vi "OpenCamera.vi"(8 "error in (no error)":errorcluster, 10 "Camera ID":string, 11 "ZWO_ASI in":refnum<class "ZWO_ASI.lvclass">) -> (0 "error out":errorcluster, 3 "ZWO_ASI out":refnum<class "ZWO_ASI.lvclass">)   [LabVIEW 2023, in "ZWO_ASI.lvlib" / "ZWO_ASI.lvclass"]
uses:
  ZWO_ASI.lvclass
  ZWO_ASI.lvclass/ZWO_ASI.ctl
  <userlib>/ASICamera2_no_err/ASICamera2_no_err.lvlib
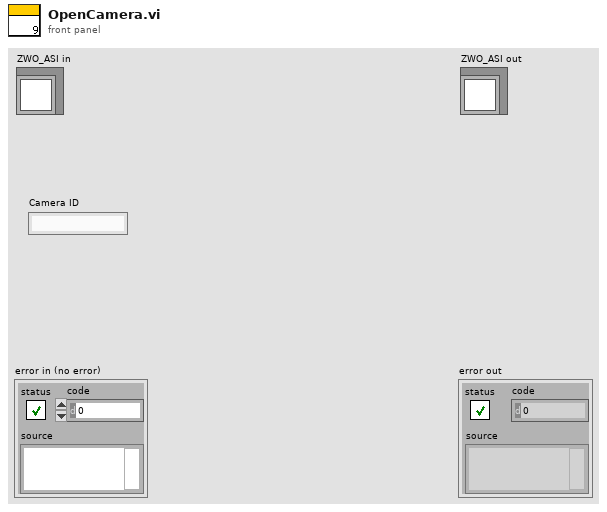
[diagram p1: front panel]
types:
  T1 = cluster{"Name[0]":i8, "Name[1]":i8, "Name[2]":i8, "Name[3]":i8, "Name[4]":i8, "Name[5]":i8, "Name[6]":i8, "Name[7]":i8, "Name[8]":i8, "Name[9]":i8, "Name[10]":i8, "Name[11]":i8, "Name[12]":i8, "Name[13]":i8, "Name[14]":i8, "Name[15]":i8, "Name[16]":i8, "Name[17]":i8, "Name[18]":i8, "Name[19]":i8, "Name[20]":i8, "Name[21]":i8, "Name[22]":i8, "Name[23]":i8, "Name[24]":i8, "Name[25]":i8, "Name[26]":i8, "Name[27]":i8, "Name[28]":i8, "Name[29]":i8, "Name[30]":i8, "Name[31]":i8, "Name[32]":i8, "Name[33]":i8, "Name[34]":i8, "Name[35]":i8, "Name[36]":i8, "Name[37]":i8, "Name[38]":i8, "Name[39]":i8, "Name[40]":i8, "Name[41]":i8, "Name[42]":i8, "Name[43]":i8, "Name[44]":i8, "Name[45]":i8, "Name[46]":i8, "Name[47]":i8, "Name[48]":i8, "Name[49]":i8, "Name[50]":i8, "Name[51]":i8, "Name[52]":i8, "Name[53]":i8, "Name[54]":i8, "Name[55]":i8, "Name[56]":i8, "Name[57]":i8, "Name[58]":i8, "Name[59]":i8, "Name[60]":i8, "Name[61]":i8, "Name[62]":i8, "Name[63]":i8, "CameraID":i32, "MaxHeight":i32, "MaxWidth":i32, "IsColorCam":u32, "BayerPattern":u32, "SupportedBins[0]":i32, "SupportedBins[1]":i32, "SupportedBins[2]":i32, "SupportedBins[3]":i32, "SupportedBins[4]":i32, "SupportedBins[5]":i32, "SupportedBins[6]":i32, "SupportedBins[7]":i32, "SupportedBins[8]":i32, "SupportedBins[9]":i32, "SupportedBins[10]":i32, "SupportedBins[11]":i32, "SupportedBins[12]":i32, "SupportedBins[13]":i32, "SupportedBins[14]":i32, "SupportedBins[15]":i32, "SupportedVideoFormat[0]":u32, "SupportedVideoFormat[1]":u32, "SupportedVideoFormat[2]":u32, "SupportedVideoFormat[3]":u32, "SupportedVideoFormat[4]":u32, "SupportedVideoFormat[5]":u32, "SupportedVideoFormat[6]":u32, "SupportedVideoFormat[7]":u32, "@dummy control@":i8, "@dummy control@":i8, "@dummy control@":i8, "@dummy control@":i8, "PixelSize":dbl, "MechanicalShutter":u32, "ST4Port":u32, "IsCoolerCam":u32, "IsUSB3Host":u32, "IsUSB3Camera":u32, "ElecPerADU":sgl, "Unused[0]":i8, "Unused[1]":i8, "Unused[2]":i8, "Unused[3]":i8, "Unused[4]":i8, "Unused[5]":i8, "Unused[6]":i8, "Unused[7]":i8, "Unused[8]":i8, "Unused[9]":i8, "Unused[10]":i8, "Unused[11]":i8, "Unused[12]":i8, "Unused[13]":i8, "Unused[14]":i8, "Unused[15]":i8, "Unused[16]":i8, "Unused[17]":i8, "Unused[18]":i8, "Unused[19]":i8, "Unused[20]":i8, "Unused[21]":i8, "Unused[22]":i8, "Unused[23]":i8}
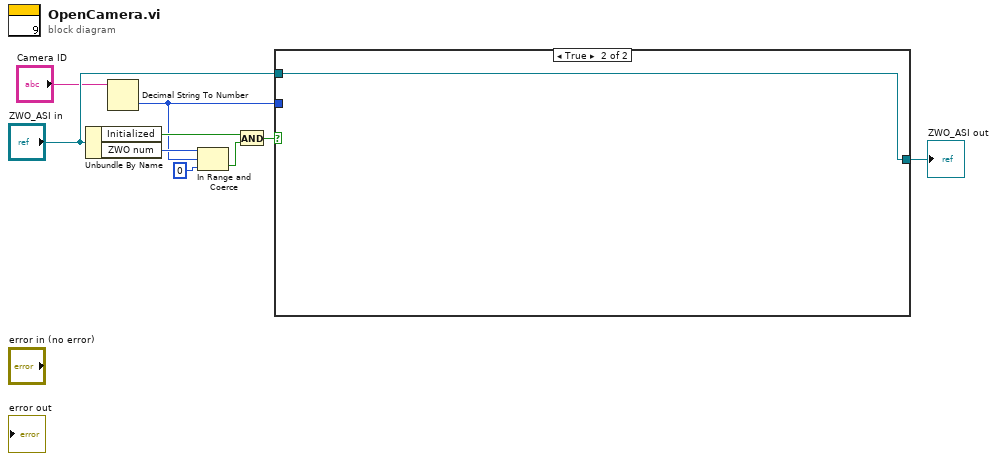
[diagram p0: block diagram]
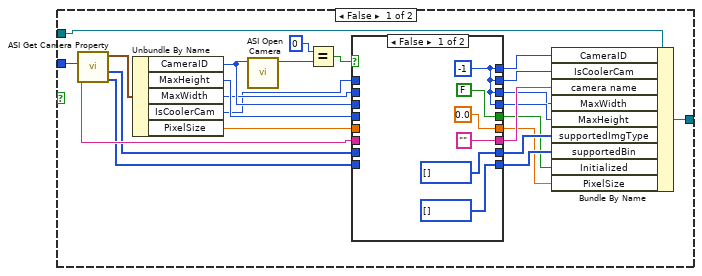
[diagram p2: hidden frame]
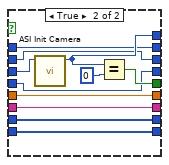
[diagram p3: hidden frame]
diagram:
  n1 = Unbundle By Name("ZWO_ASI in") -> ("Initialized"=w3:bool, "ZWO num"=w6:i32)
  n2 = Decimal String To Number(string="Camera ID") -> (number=w1:i32)  [unwired: 2 in, 1 out]
  n3 = In Range and Coerce(upper limit=w6, x=w1, lower limit=0) -> (In Range?=w4:bool)  [unwired: 1 out]
  n4 = And(x=w3, y=w4) -> (x .and. y?=w2:bool)
  n5 = case shown="True" w2 {
    tunnel: w1 -> [w28 _]
    tunnel: "ZWO_ASI in" -> [w27 w51]
    tunnel: [w26 w51] -> w8
    frame False {
      n6 = call <userlib>:"ASI Get Camera Property.vi"("iCameraIndex"=w28) -> ("supportedBin"=w19:i8[], "supportedImgType"=w18:i8[], "pASICameraInfo out"=w31:T1, "cameraName"=w23:string)  [unwired: 6 in, 1 out]
      n7 = Unbundle By Name(w31) -> ("CameraID"=w29:i32, "MaxHeight"=w21:i32, "MaxWidth"=w14:i32, "IsCoolerCam"=w13:u32, "PixelSize"=w11:dbl)
      n8 = call <userlib>:"ASI Open Camera.vi"("iCameraID"=w29) -> ("function return"=w33:i32)  [unwired: 10 in]
      n9 = Equal?(x=0, y=w33) -> (x = y?=w30:bool)
      n10 = case shown="False" w30 {
        tunnel: [FALSE w49] -> w12
        tunnel: w29 -> [_ w48]
        tunnel: [w38 w47] -> w25
        tunnel: [w38 w41] -> w24
        tunnel: w23 -> [_ w46]
        tunnel: ["" ("cameraName") w46] -> w22
        tunnel: w21 -> [_ w43]
        tunnel: [i8[] [] ("supportedBin") w45] -> w20
        tunnel: w19 -> [_ w45]
        tunnel: w18 -> [_ w44]
        tunnel: [i8[] [] ("supportedImgType") w44] -> w17
        tunnel: [w38 w43] -> w16
        tunnel: [w38 w42] -> w15
        tunnel: w14 -> [_ w42]
        tunnel: w13 -> [_ w41]
        tunnel: w11 -> [_ w40]
        tunnel: [0.0 ("PixelSize") w40] -> w10
        frame False {
          w38 = -1 ("function return")
        }
        frame True {
          n11 = call <userlib>:"ASI Init Camera.vi"("iCameraID"=w48) -> ("function return"=w47:i32)  [unwired: 10 in]
          n12 = Equal?(x=w47, y=0 ("x")) -> (x = y?=w49:bool)
        }
      }
      n13 = Bundle By Name(cluster=w27, "CameraID"=w25, "IsCoolerCam"=w24, "camera name"=w22, "MaxWidth"=w15, "MaxHeight"=w16, "supportedImgType"=w17, "supportedBin"=w20, "Initialized"=w12, "PixelSize"=w10) -> (w26:refnum<class "ZWO_ASI.lvclass">)
    }
    frame True {
    }
  }
  "ZWO_ASI out" <- w8
